vi "KeDSO High Resolution Parameters.vi"(8 "error in":errorcluster, 11 "keysight dso":T1={"VISA"="", "channels"=[], "bw limit [Hz]"=0.0, "resolution"=enum."Basic", "trig noise reject"=enum."Normal", "N"=0, "trigger config"={"trigger source"=enum."Immediate", "trigger slope"=enum."Negative", "level [V]"=0.0, "hysteresis [V]"=0.001, "pre-trig [%]"=50}, "fs [Hz]"=0.0, "timeout stop"=timestamp(0 s since 1904-01-01), "waiting for opc"=FALSE, "fetch offset [smpl]"=0, "abs timestamp"=timestamp(0 s since 1904-01-01), "ranges [V]"=[], "decimation"=0.0, "ext ref"=FALSE, "emulate aperture"=FALSE, "model"=enum."DSO91304"} {"bw limit [Hz]" format="%#_6p"; "channels"."Offset [V]" format="%#_6p"; "channels"."Range [Vpk]" min=0.0 format="%#_6p"; "channels"."Channel" min=1}) -> (0 "error out":errorcluster, 1 "Resolution":i32(ring) items=["Auto", "Bits 9", "Bits 10", "Bits 11", "Bits 12", "Fixed 11", "Fixed 12", "Fixed 13", "Fixed 14", "Fixed 15", "Fixed 16"], 2 "Acquisition Type":i32(ring) items=["Normal", "Peak Detect", "High Resolution"], 3 "keysight dso out":T1={"VISA"="", "channels"=[], "bw limit [Hz]"=0.0, "resolution"=enum."Basic", "trig noise reject"=enum."Normal", "N"=0, "trigger config"={"trigger source"=enum."Immediate", "trigger slope"=enum."Negative", "level [V]"=0.0, "hysteresis [V]"=0.001, "pre-trig [%]"=50}, "fs [Hz]"=0.0, "timeout stop"=timestamp(0 s since 1904-01-01), "waiting for opc"=FALSE, "fetch offset [smpl]"=0, "abs timestamp"=timestamp(0 s since 1904-01-01), "ranges [V]"=[], "decimation"=0.0, "ext ref"=FALSE, "emulate aperture"=FALSE, "model"=enum."DSO91304"} {"bw limit [Hz]" format="%#_6p"; "channels"."Offset [V]" format="%#_6p"; "channels"."Range [Vpk]" min=0.0 format="%#_6p"; "channels"."Channel" min=1}, 4 "fixed bits?":bool, 5 "fs info valid?":bool, 6 "fs list [Hz]":dbl[](array[numeric]))   [LabVIEW 2020]
doc: "Gets parameters of high res mode (bits, sample rates, etc.)"
uses:
  KeDSO session.ctl
  KeDSO Virtual Channel.ctl
  KeDSO High Resolution Mode.ctl
  KeDSO Trigger Setup.ctl
  KeDSO Trigger Source.ctl
  Public/Utility/DSO type.ctl
  Agilent 90000 Series.lvlib
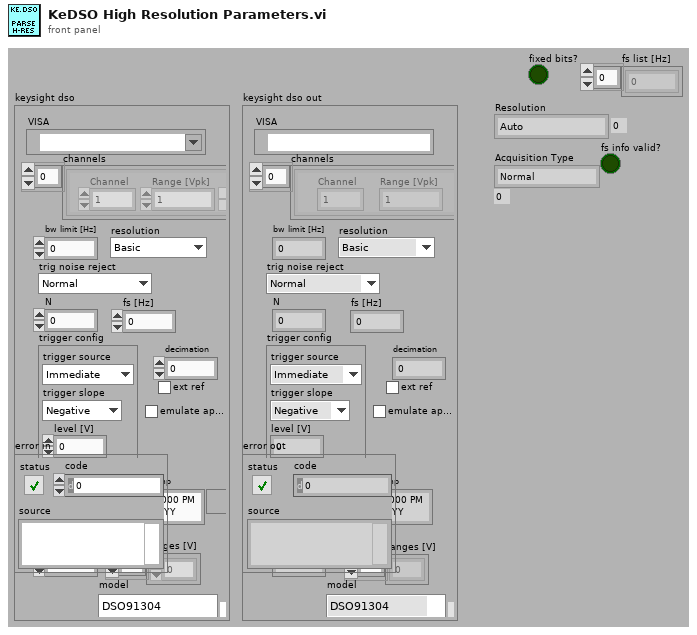
[diagram p1: front panel]
types:
  T1 = typedef "KeDSO session.ctl" = cluster{"VISA":refnum<visa-resource-name>, "channels":T2[], "bw limit [Hz]":dbl, "resolution":T3, "trig noise reject":enum16{"Normal", "High Sensitivity"}, "N":i64, "trigger config":T4, "fs [Hz]":dbl, "timeout stop":timestamp, "waiting for opc":bool, "fetch offset [smpl]":i64, "abs timestamp":timestamp, "ranges [V]":dbl[], "decimation":dbl, "ext ref":bool, "emulate aperture":bool, "model":T6}
  T2 = typedef "KeDSO Virtual Channel.ctl" = cluster{"Channel":i32, "Range [Vpk]":dbl, "btn clr":bool, "btn up":bool, "btn down":bool, "Offset [V]":dbl, "Coupling":enum16{"DC", "DC50", "AC", "LFR1"}, "bw limit enab":bool}
  T3 = typedef "KeDSO High Resolution Mode.ctl" = enum16{"Basic", "High-res AUTO", "Min. 9-bits", "Min. 10-bits", "Min. 11-bits", "Min. 12-bits", "Fixed 11-bits", "Fixed 12-bits", "Fixed 13-bits", "Fixed 14-bits", "Fixed 15-bits", "Fixed 16-bits"}
  T4 = typedef "KeDSO Trigger Setup.ctl" = cluster{"trigger source":T5, "trigger slope":enum16{"Negative", "Positive", "Either"}, "level [V]":dbl, "hysteresis [V]":dbl, "pre-trig [%]":i32}
  T5 = typedef "KeDSO Trigger Source.ctl" = enum16{"Immediate", "Level", "AUX"}
  T6 = typedef "Agilent 90000 Series.lvlib/DSO type.ctl" = enum16{"DSO91304", "DSO91204", "DSO90804", "DSO90604", "DSO90404", "DSO90254", "DSA91304", "DSA91204", "DSA90804", "DSA90604", "DSA90404", "DSA90254", "DSO9104", "DSO9254", "DSO9404", "MSO9104", "MSO9254", "MSO9404", "MSO9064", "DSO9064", "DSOX91604", "DSOX92004", "DSOX92504", "DSOX92804", "DSOX93204", "DSO93004", "DSO9024H", "DSO9054H", "DSO9104H", "DSO9204H", "DSOS054A", "DSOS104A", "DSOS204A", "DSOS254A", "DSOS404A", "DSOS604A", "DSOS804A", "MSOS054A", "MSOS104A", "MSOS204A", "MSOS254A", "MSOS404A", "MSOS604A", "MSOS804A", "DSAX96204Q", "DSOX96204Q", "DSAX95004Q", "DSOX95004Q", "DSAX93304Q", "DSOX93304Q", "DSAX92504Q", "DSOX92504Q", "DSAX92004Q", "DSOX92004Q"}
  T7 = cluster{"resolution":T3, "bits":i32, "fixed":bool}[]
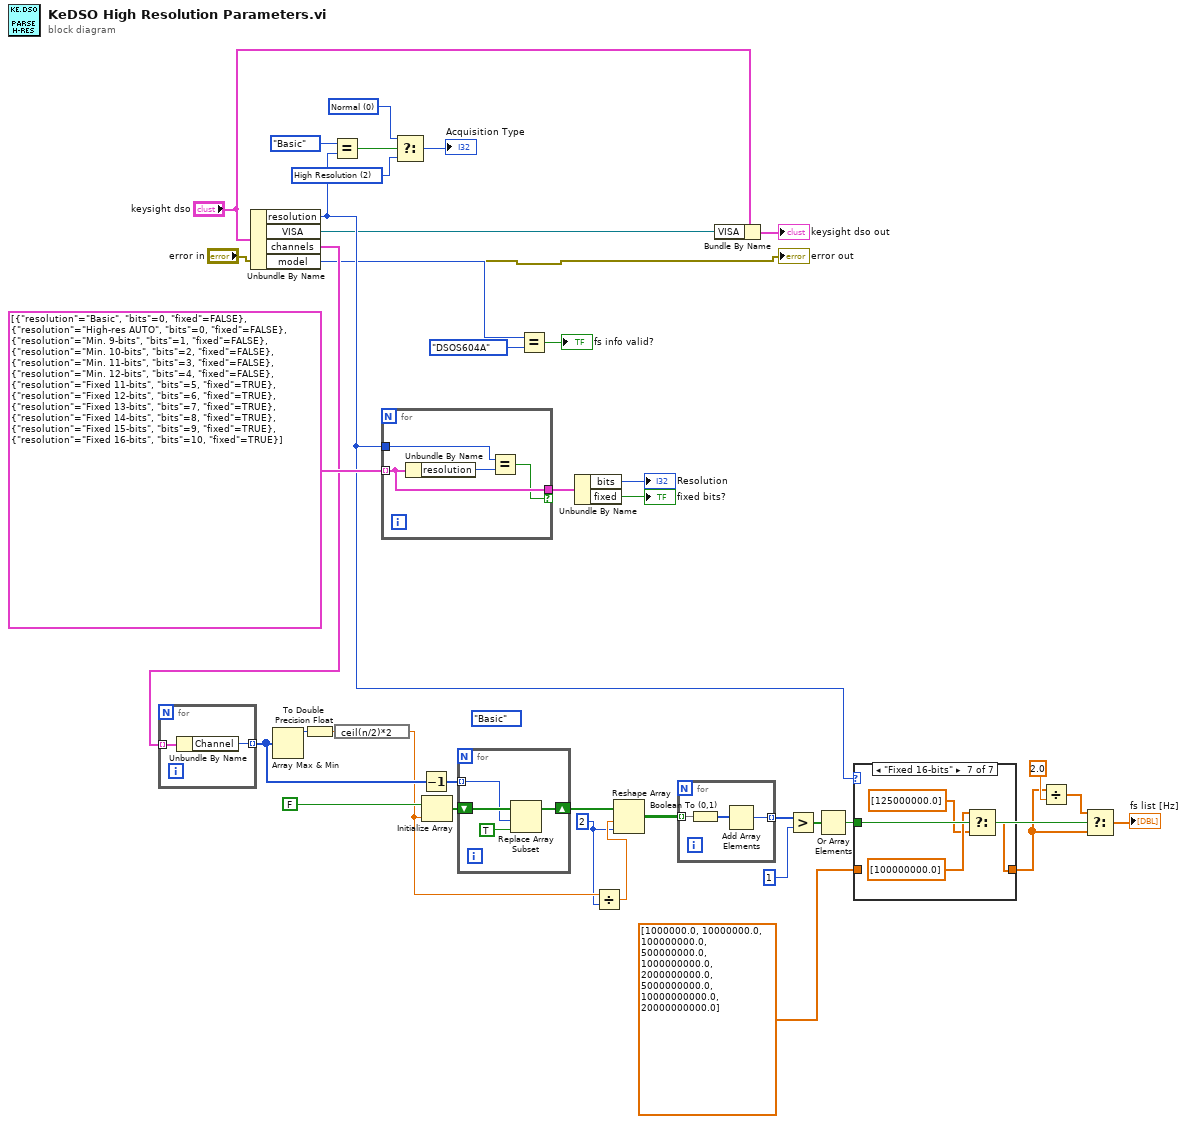
[diagram p0: block diagram]
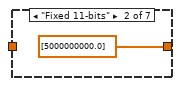
[diagram p3: hidden frame]
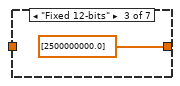
[diagram p4: hidden frame]
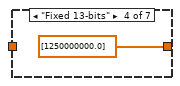
[diagram p5: hidden frame]
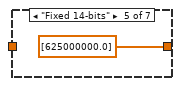
[diagram p6: hidden frame]
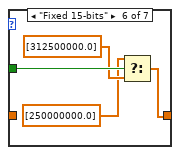
[diagram p7: hidden frame]
diagram:
  w17 = 2 ("dimension size")
  (unwired) KeDSO_High_Resolution_Mode."Basic" ("keysight dso.resolution")
  w33 = 2 items=["Normal", "Peak Detect", "High Resolution"] ("Acquisition Type (0: Normal)")
  w34 = 0 items=["Normal", "Peak Detect", "High Resolution"] ("Acquisition Type (0: Normal)")
  n1 = Unbundle By Name("keysight dso") -> ("resolution"=w8:T3, "VISA"=w3:refnum<visa-resource-name>, "channels"=w7:T2[], "model"=w2:T6)
  n2 = for {
    tunnel: w7 -> [w40] mode=indexing
    tunnel: [w39] -> w24 mode=indexing
    n3 = Unbundle By Name(w40) -> ("Channel"=w39:i32)
  }
  n4 = Array Max & Min(array=w24) -> (max value=w27:i32)  [unwired: 3 out]
  n5 = To Double Precision Float(number=w27) -> (double precision float=w21:dbl)
  n6 = Equal?(x=KeDSO_High_Resolution_Mode."Basic", y=w8) -> (x = y?=w35:bool)
  n7 = expression code="ceil(n/2)*2"(w21) -> (w20:dbl)
  n8 = for {
    tunnel: T7 [{"resolution"=enum."Basic", "bits"=0, "fixed"=FALSE}, {"resolution"=enum."High-res AUTO", "bits"=0, "fixed"=FALSE}, {"resolution"=enum."Min. 9-bits", "bits"=1, "fixed"=FALSE}, {"resolution"=enum."Min. 10-bits", "bits"=2, "fixed"=FALSE}, {"resolution"=enum."Min. 11-bits", "bits"=3, "fixed"=FALSE}, {"resolution"=enum."Min. 12-bits", "bits"=4, "fixed"=FALSE}, {"resolution"=enum."Fixed 11-bits", "bits"=5, "fixed"=TRUE}, {"resolution"=enum."Fixed 12-bits", "bits"=6, "fixed"=TRUE}, {"resolution"=enum."Fixed 13-bits", "bits"=7, "fixed"=TRUE}, {"resolution"=enum."Fixed 14-bits", "bits"=8, "fixed"=TRUE}, {"resolution"=enum."Fixed 15-bits", "bits"=9, "fixed"=TRUE}, {"resolution"=enum."Fixed 16-bits", "bits"=10, "fixed"=TRUE}] -> [w42] mode=indexing
    tunnel: w8 -> [w43]
    tunnel: [w42] -> w30 if=w41
    n9 = Unbundle By Name(w42) -> ("resolution"=w44:T3)
    n10 = Equal?(x=w43, y=w44) -> (x = y?=w41:bool)
  }
  n11 = Select(t=w34, s=w35, f=w33) -> (s? t:f=→"Acquisition Type":i32)
  n12 = Decrement(x=w24) -> (x-1=w23:i32[])
  n13 = Initialize Array(FALSE, w20) -> (w25:bool[])
  n14 = for {
    shift-right: [w47] -> w22
    shift-left: w25 -> [w48]
    tunnel: w23 -> [w45] mode=indexing
    n15 = Replace Array Subset(array=w48, new element=TRUE, index=w45) -> (w47:bool[])
  }
  n16 = Equal?(x=w2, y=DSO_type."DSOS604A") -> (x = y?=→"fs info valid?":bool)
  n17 = Unbundle By Name(w30) -> ("bits"=→"Resolution":i32, "fixed"=→"fixed bits?":bool)
  n18 = Divide(x=w20, y=w17) -> (x/y=w18:dbl)
  n19 = Reshape Array(w22, w18, w17) -> (w19:bool[][])
  n20 = for {
    tunnel: w19 -> [w51] mode=indexing
    tunnel: [w49] -> w16 mode=indexing
    n21 = Boolean To (0,1)(Boolean=w51) -> (0, 1=w50:i16[])
    n22 = Add Array Elements(numeric array=w50) -> (sum=w49:i16)
  }
  n23 = Bundle By Name(cluster="keysight dso", "VISA"=w3) -> (→"keysight dso out":T1)
  n24 = Greater?(x=w16, y=1) -> (0:w14:bool[])
  n25 = Or Array Elements(Boolean array=w14) -> (logical OR=w10:bool)
  n26 = case shown="\"Fixed 16-bits\"" w8 {
    tunnel: dbl[] [1000000.0, 10000000.0, 100000000.0, 500000000.0, 1000000000.0, 2000000000.0, 5000000000.0, 10000000000.0, 20000000000.0] -> [w52 _ _ _ _ _ _]
    tunnel: [w52 dbl[] [5000000000.0] dbl[] [2500000000.0] dbl[] [1250000000.0] dbl[] [625000000.0] w57 w61] -> w9
    tunnel: w10 -> [_ _ _ _ _ w60 w64]
    frame "Basic", Default {
    }
    frame "Fixed 11-bits" {
    }
    frame "Fixed 12-bits" {
    }
    frame "Fixed 13-bits" {
    }
    frame "Fixed 14-bits" {
    }
    frame "Fixed 15-bits" {
      n27 = Select(t=dbl[] [250000000.0], s=w60, f=dbl[] [312500000.0]) -> (s? t:f=w57:dbl[])
    }
    frame "Fixed 16-bits" {
      n28 = Select(t=dbl[] [100000000.0], s=w64, f=dbl[] [125000000.0]) -> (s? t:f=w61:dbl[])
    }
  }
  n29 = Divide(x=w9, y=2.0 ("mclk [Hz]")) -> (x/y=w13:dbl[])
  n30 = Select(t=w13, s=w10, f=w9) -> (s? t:f=→"fs list [Hz]":dbl[])
  "error out" <- "error in"
